vi "ADO Fields Item.vi"(8 "error in (no error)":errorcluster, 10 "Index":i32, 11 "Fields In":refnum<k7>) -> (0 "error out":errorcluster, 2 "Item Out":refnum<k7>, 3 "Fields Out":refnum<k7>)   [LabVIEW 2011]
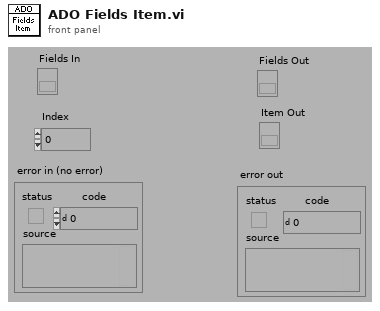
[diagram p1: front panel]
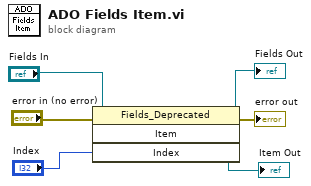
[diagram p0: block diagram]
diagram:
  n1 = invoke class="Fields_Deprecated" method="Item"(reference="Fields In", error in="error in (no error)", "Index"="Index") -> (reference out=→"Fields Out":refnum<k7>, error out=→"error out":errorcluster, "Item"=→"Item Out":refnum<k7>)  [unwired: 1 in, 1 out]
